vi "Initialize1.vi"   [LabVIEW 2020]
uses:
  FlatField Status.ctl
  FlatFieldUI/FlatFieldUI.lvclass
  Displayer/Displayer/FlatField Method.ctl
types:
  T1 = typedef "FlatField.lvlib/FlatFieldUI.lvlib/FlatFieldUI.lvclass/FlatField Method.ctl" = i32
  T2 = typedef "Image Type" = u32
  T3 = typedef "FlatField.lvlib/FlatFieldUI.lvlib/FlatFieldUI.lvclass/FlatField Status.ctl" = i32
  T4 = typedef "IMAQ Image.ctl" = refnum<image>
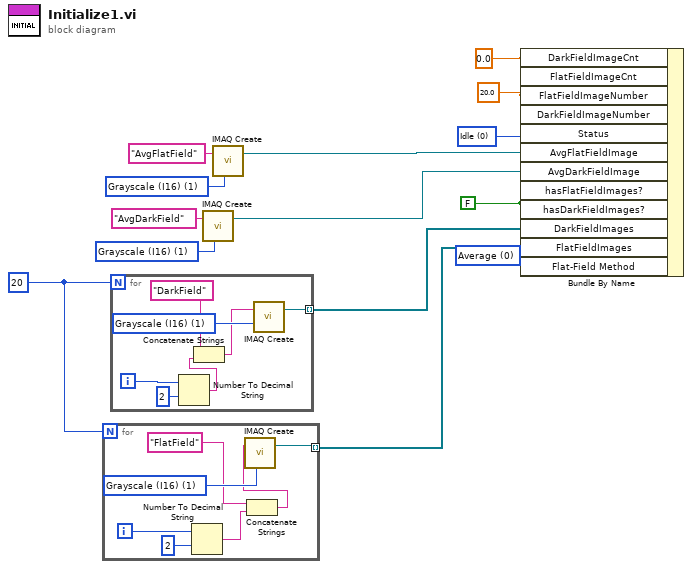
[diagram p0: block diagram]
diagram:
  w1 = T1 0 items=["Average", "Median"] ("Flat-Field Method")
  w4 = 20
  w5 = FALSE ("hasFlatFieldImages?")
  w8 = T2 1 items=["Grayscale (U8)", "Grayscale (I16)", "Grayscale (SGL)", "Complex (CSG)", "RGB (U32)", "HSL (U32)", "RGB (U64)", "Grayscale (U16)"] ("Image Type")
  w9 = T2 1 items=["Grayscale (U8)", "Grayscale (I16)", "Grayscale (SGL)", "Complex (CSG)", "RGB (U32)", "HSL (U32)", "RGB (U64)", "Grayscale (U16)"] ("Image Type")
  w12 = 0.0 ("DarkFieldImageCnt")
  w13 = 20.0 ("FieldFieldImageNumber")
  w14 = T3 0 items=["Idle", "Taking DarkField Images", "Taking FlatField Image", "Doing FlatField", ""] ("Flat-Field Status")
  n1 = for {
    N: w4 -> [_]
    tunnel: [w15] -> w2 mode=indexing
    i -> [w20]
    w21 = T2 1 items=["Grayscale (U8)", "Grayscale (I16)", "Grayscale (SGL)", "Complex (CSG)", "RGB (U32)", "HSL (U32)", "RGB (U64)", "Grayscale (U16)"] ("Image Type")
    n2 = Number To Decimal String(number=w20, width (-)=i16 2) -> (decimal integer string=w17:string)
    n3 = Concatenate Strings("FlatField" ("Image Name"), w17) -> (w16:string)
    n4 = call "IMAQ Create"("Image Name"=w16, "Image Type"=w21) -> ("New Image"=w15:T4)  [unwired: 3 in, 1 out]
  }
  n5 = for {
    N: w4 -> [_]
    tunnel: [w22] -> w3 mode=indexing
    i -> [w27]
    w28 = T2 1 items=["Grayscale (U8)", "Grayscale (I16)", "Grayscale (SGL)", "Complex (CSG)", "RGB (U32)", "HSL (U32)", "RGB (U64)", "Grayscale (U16)"] ("Image Type")
    n6 = Number To Decimal String(number=w27, width (-)=i16 2) -> (decimal integer string=w25:string)
    n7 = Concatenate Strings("DarkField" ("Image Name"), w25) -> (w23:string)
    n8 = call "IMAQ Create"("Image Name"=w23, "Image Type"=w28) -> ("New Image"=w22:T4)  [unwired: 3 in, 1 out]
  }
  n9 = call "IMAQ Create"("Image Name"="AvgDarkField", "Image Type"=w8) -> ("New Image"=w6:T4)  [unwired: 3 in, 1 out]
  n10 = call "IMAQ Create"("Image Name"="AvgFlatField", "Image Type"=w9) -> ("New Image"=w11:T4)  [unwired: 3 in, 1 out]
  n11 = Bundle By Name("DarkFieldImageCnt"=w12, "FlatFieldImageCnt"=w12, "FlatFieldImageNumber"=w13, "DarkFieldImageNumber"=w13, "Status"=w14, "AvgFlatFieldImage"=w11, "AvgDarkFieldImage"=w6, "hasFlatFieldImages?"=w5, "hasDarkFieldImages?"=w5, "DarkFieldImages"=w3, "FlatFieldImages"=w2, "Flat-Field Method"=w1) -> ()  [unwired: 1 in, 1 out]
